vi "Configure Offset Compensation.vi"(7 "Enable Offset Compensation (T: Enable)":bool=TRUE, 8 "error in (no error)":errorcluster, 11 "VISA resource name":refnum<visa-resource-name>) -> (0 "error out":errorcluster, 3 "VISA resource name out":refnum<visa-resource-name>)   [LabVIEW 2013, in "Agilent 34401.lvlib"]
doc: "Enables or disables offset compensation for resistance measurements.\n\n<B>Note:</B>\n\nThis VI only applies to the Agilent 34410/34411 models."
uses:
  Agilent 34401.lvlib
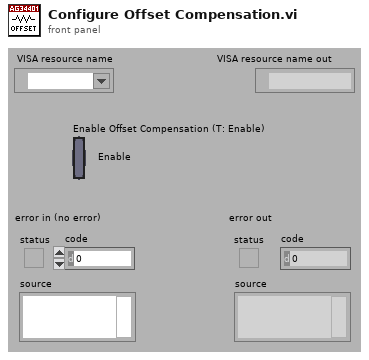
[diagram p1: front panel]
types:
  T1 = typedef "Agilent 34401.lvlib/Extended User Data.ctl" = cluster{"Trigger Source":u16, "Math Storage":u16, "Agilent Model":i32}
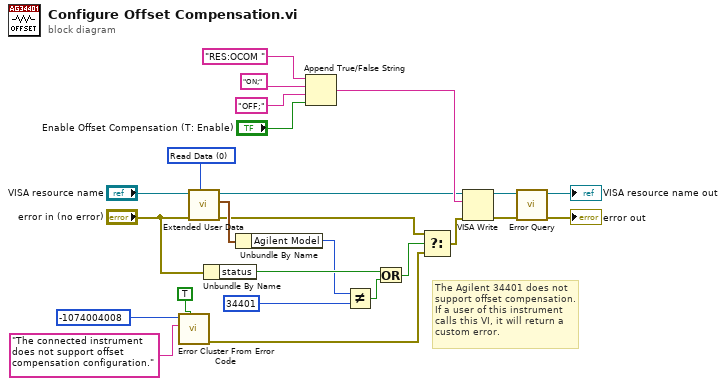
[diagram p0: block diagram]
diagram:
  w6 = u16 0 items=["Read Data", "Write Data", "Dispose of Data"] ("Action")
  # "The Agilent 34401 does not support offset compensation. If a user of this instrument calls this VI, it will return a custom error."
  n1 = call <vilib>:"Error Cluster From Error Code.vi"("show call chain? (False)"=TRUE, "error message (\"\")"="The connected instrument does not support offset compensation configuration." ("Source (VI Name)"), "error code (0)"=-1074004008 ("Code")) -> ("error out"=w13:errorcluster)  [unwired: 6 in]
  n2 = call "Extended User Data.vi"("Action"=w6, "Error In (no error)"="error in (no error)", "VISA resource name in"="VISA resource name") -> ("Error Out"=w2:errorcluster, "User Data Out"=w7:T1, "VISA resource name out"=w3:refnum<visa-resource-name>)  [unwired: 6 in]
  n3 = Unbundle By Name("error in (no error)") -> ("status"=w10:bool)
  n4 = Unbundle By Name(w7) -> ("Agilent Model"=w1:i32)
  n5 = Append True/False String(1:"Enable Offset Compensation (T: Enable)", 2:"OFF;", 3:"ON;", 4:"RES:OCOM " ("initial string")) -> (0:w14:string)
  n6 = Not Equal?(x=w1, y=u32 34401 ("x")) -> (x != y?=w9:bool)
  n7 = Or(x=w10, y=w9) -> (x .or. y?=w8:bool)
  n8 = Select(t=w2, s=w8, f=w13) -> (s? t:f=w12:errorcluster)
  n9 = VISA Write(VISA resource name=w3, write buffer=w14, error in (no error)=w12) -> (VISA resource name out=w23:refnum<visa-resource-name>, error out=w22:errorcluster)  [unwired: 1 out]
  n10 = call "Error Query.vi"("error in (no error)"=w22, "VISA resource name"=w23) -> ("error out"=→"error out":errorcluster, "VISA resource name out"=→"VISA resource name out":refnum<visa-resource-name>)  [unwired: 6 in, 2 out]
